vi "LED Test.vi"() -> ()   [LabVIEW 2014]
panel:
  in  "stop":bool
  in  "Camera":bool
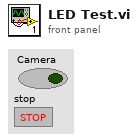
[diagram p1: front panel]
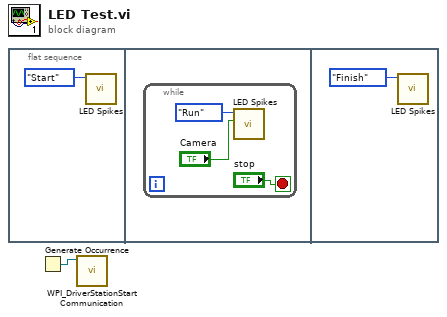
[diagram p0: block diagram]
diagram:
  n1 = flat-sequence {
    frame #0 {
      n2 = call "LED Spikes.vi"("Mode"=enum8{"Start", "Run", "Finish"}."Start") -> ()  [unwired: 3 in]
    }
    frame #1 {
      n3 = while {
        stop <- "stop" stop-if-true
        n4 = call "LED Spikes.vi"("Camera LED ON/OFF"="Camera", "Mode"=enum8{"Start", "Run", "Finish"}."Run") -> ()  [unwired: 2 in]
      }
    }
    frame #2 {
      n5 = call "LED Spikes.vi"("Mode"=enum8{"Start", "Run", "Finish"}."Finish") -> ()  [unwired: 3 in]
    }
  }
  n6 = Generate Occurrence() -> (w1:refnum<k4>)
  n7 = call <vilib>:"WPI_DriverStationStart Communication.vi"("occurrence"=w1) -> ()  [unwired: 11 in]
